vi "Change Icon Template.vi"(8 "error in (no error)":errorcluster, 11 "VI Reference In":refnum<vi>) -> (0 "error out":errorcluster, 3 "VI Reference Out":refnum<vi>)   [LabVIEW 2015]
uses:
  <vilib>/picture/picture.llb/Draw True-Color Pixmap.vi
panel:
  out "New Icon":picture
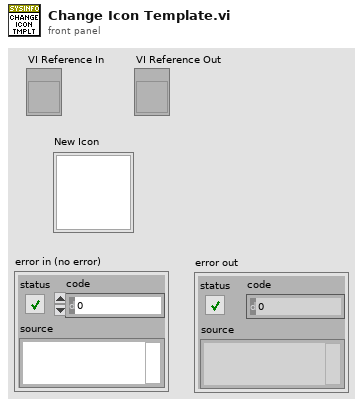
[diagram p1: front panel]
types:
  T1 = cluster{"left":i16, "top":i16, "right":i16, "bottom":i16}
  T2 = typedef "imagedata.ctl" = cluster{"image type":i32, "image depth":i32, "image":u8[], "mask":u8[], "colors":u32[], "Rectangle":cluster{"left":i16, "top":i16, "right":i16, "bottom":i16}}
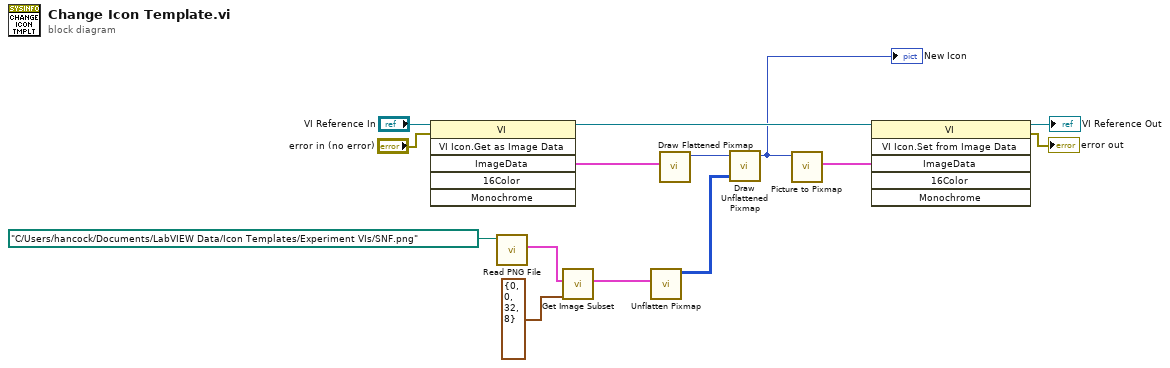
[diagram p0: block diagram]
diagram:
  n1 = invoke class="VI" method="VI Icon.Get as Image Data"(reference="VI Reference In", error in="error in (no error)") -> (reference out=w9:refnum<vi>, "ImageData"=w13:T2)  [unwired: 4 in, 4 out]
  n2 = call <vilib>:"Read PNG File.vi"("path to PNG file"=path "C:/Users/hancock/Documents/LabVIEW Data/Icon Templates/Experiment VIs/SNF.png") -> ("image data"=w2:T2)  [unwired: 8 in, 2 out]
  n3 = call <vilib>:"Get Image Subset.vi"("subset rect"=T1 {"left"=0, "top"=0, "right"=32, "bottom"=8}, "image data"=w2) -> ("image subset"=w1:T2)  [unwired: 4 in, 1 out]
  n4 = call <vilib>:"Unflatten Pixmap.vi"("image data"=w1) -> ("24-bit pixmap"=w11:u32[][])  [unwired: 4 in, 6 out]
  n5 = call <vilib>:"Draw Flattened Pixmap.vi"("image data"=w13) -> ("new picture"=w12:picture)  [unwired: 8 in]
  n6 = call-poly <vilib>:"Draw Unflattened Pixmap.vi"("picture"=w12, "data (RGB format)"=w11) -> ("new picture"=w8:picture)  [unwired: 7 in]
  "New Icon" <- w8
  n7 = call <vilib>:"Picture to Pixmap.vi"("picture"=w8) -> ("image data"=w7:T2)  [unwired: 9 in, 1 out]
  n8 = invoke class="VI" method="VI Icon.Set from Image Data"(reference=w9, "ImageData"=w7) -> (reference out=→"VI Reference Out":refnum<vi>, error out=→"error out":errorcluster)  [unwired: 4 in, 4 out]
